vi "Bind to Name - Error Input - Returns Same Error.vi"() -> ()   [LabVIEW 2017, in "JSON Serializable Binder Tests.lvlib"]
uses:
  JSON Serializable Binder Tests.lvlib
  JSON Serializable Binder/JSON Serializable Binder.lvclass
  <vilib>/Utility/error.llb/Error Cluster From Error Code.vi
  <vilib>/addons/_JKI Toolkits/Caraya/classes/Assert/Assert Equal Value_Variant.vi
  <vilib>/ErrorRing/Error Ring.xnode
  <vilib>/addons/_JKI Toolkits/Caraya/classes/Test/Test.lvclass
  <vilib>/addons/_JKI Toolkits/Caraya/classes/Assert/Assert.lvclass
panel:
  out "error out":errorcluster
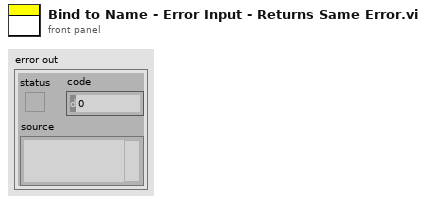
[diagram p1: front panel]
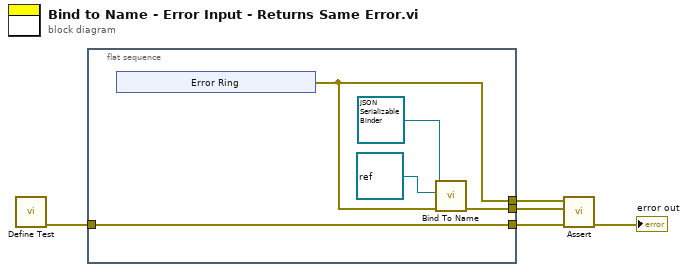
[diagram p0: block diagram]
diagram:
  n1 = call <vilib>:"Define Test.vi"() -> ("error out"=w2:errorcluster)  [unwired: 11 in]
  n2 = flat-sequence {
    tunnel: [w10] -> w5
    tunnel: [w9] -> w4
    tunnel: [w8] -> w3
    tunnel: w2 -> [w8]
    frame #0 {
      n3 = xnode "Error Ring"() -> ("error out"=w9:errorcluster)
      n4 = call-dynamic "Bind To Name.vi"("error in (no error)"=w9, "Type"=refnum<class> refnum, "JSON Serializable Binder in"=refnum<class "JSON Serializable Binder.lvclass"> refnum ("JSON Serializable Binder.lvclass")) -> ("error out"=w10:errorcluster)  [unwired: 6 in, 2 out]
    }
  }
  n5 = call-poly <vilib>:"Assert.vi"("error in (no error)"=w3, "Y"=w5, "X"=w4) -> ("error out"=→"error out":errorcluster)  [unwired: 8 in]
